vi "AWS-S3-SynchronousUpload.vi"(0 "AWS-S3-API":refnum<class "AWS-S3-API.lvclass">, 5 "Object Key":string, 7 "Object Bucket":string, 9 "Content Body":string, 11 "error in":errorcluster, 12 "Metadata":T1[](array[typedef])) -> (4 "AWS-S3-API out":refnum<class "AWS-S3-API.lvclass">, 15 "error out":errorcluster)   [LabVIEW 2012, in "AWS-S3-API.lvclass"]
uses:
  AWS-S3-API.lvclass
  AWS Shared/AWS-Shared-MetadataKeyValuePair.ctl
  C:/Users/Jack/repo/visualize/Dependencies/aws/AWS-SDK/AWSSDK.dll
  AWS-SDK/AWSSDK.dll
panel:
  # "Inputs"
  # "Outputs"
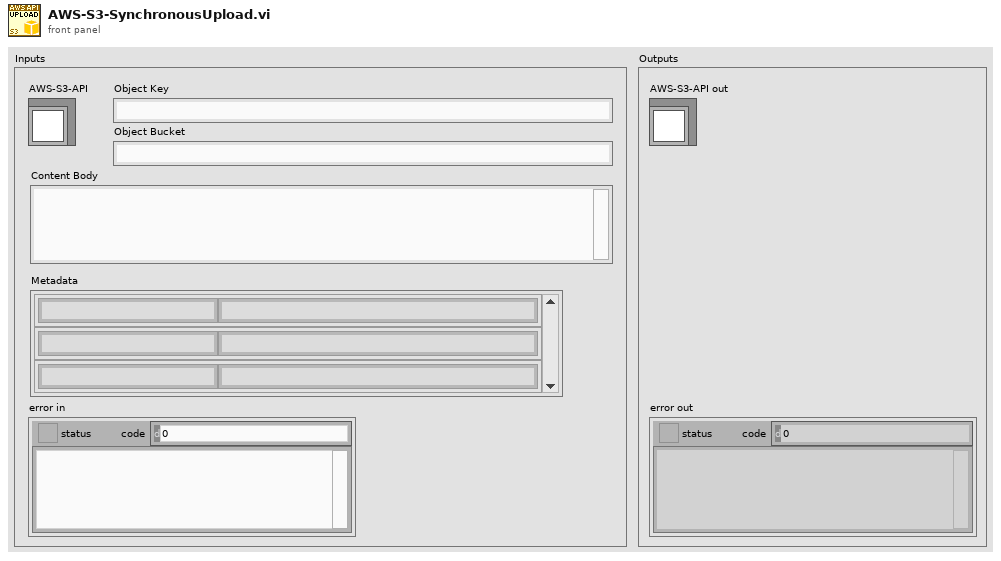
[diagram p1: front panel]
types:
  T1 = typedef "AWS-Shared-MetadataKeyValuePair.ctl" = cluster{"Key":string, "Value":string}
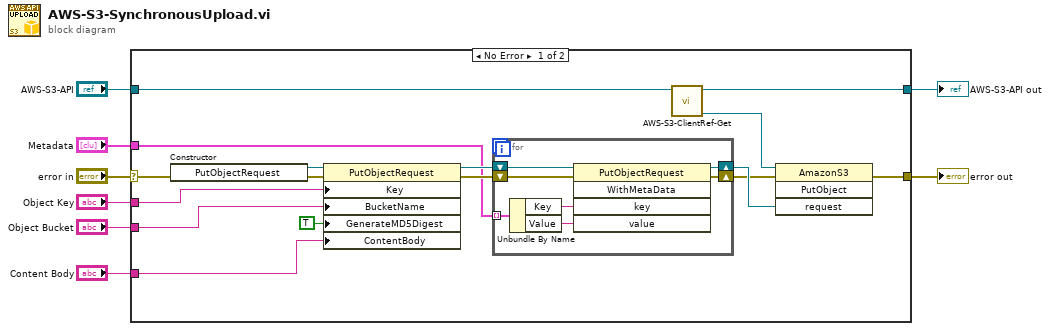
[diagram p0: block diagram]
diagram:
  n1 = case shown="No Error" "error in" {
    selector: "error in" -> [w16 w33]
    tunnel: [w12 w33] -> w8
    tunnel: [w10 w32] -> w6
    tunnel: "AWS-S3-API" -> [w11 w32]
    tunnel: "Content Body" -> [w15 _]
    tunnel: "Object Key" -> [w23 _]
    tunnel: "Object Bucket" -> [w22 _]
    tunnel: "Metadata" -> [w17 _]
    frame No Error {
      n2 = constructor class="PutObjectRequest"(error in=w16) -> (reference out=w20:refnum<k24>, error out=w24:errorcluster)  [unwired: 2 in, 1 out]
      n3 = property class="PutObjectRequest"(reference=w20, error in=w24, "Key"=w23, "BucketName"=w22, "GenerateMD5Digest"=TRUE, "ContentBody"=w15) -> (reference out=w19:refnum<k24>, error out=w18:errorcluster)
      n4 = for {
        shift-right: [w28] -> w14
        shift-left: w19 -> [w31]
        shift-right: [w29] -> w13
        shift-left: w18 -> [w30]
        tunnel: w17 -> [w27] mode=indexing
        n5 = Unbundle By Name(w27) -> ("Key"=w26:string, "Value"=w25:string)
        n6 = invoke class="PutObjectRequest" method="WithMetaData"(reference=w31, error in=w30, "key"=w26, "value"=w25) -> (reference out=w28:refnum<k24>, error out=w29:errorcluster)  [unwired: 1 in, 3 out]
      }
      n7 = call "AWS-S3-ClientRef-Get.vi"("AWS-S3-API"=w11) -> ("S3 Client ref"=w9:refnum<k24>, "AWS-S3-API out"=w10:refnum<class "AWS-S3-API.lvclass">)  [unwired: 9 in]
      n8 = invoke class="AmazonS3" method="PutObject"(reference=w9, error in=w13, "request"=w14) -> (error out=w12:errorcluster)  [unwired: 1 in, 3 out]
    }
    frame Error {
    }
  }
  "error out" <- w8
  "AWS-S3-API out" <- w6
